vi "Get busy.vi"(8 "error in (no error)":errorcluster, 11 "Retiga in":refnum<class "Retiga.lvclass">) -> (0 "error out":errorcluster, 2 "busy?":bool, 3 "Retiga out":refnum<class "Retiga.lvclass">)   [LabVIEW 2012, in "Retiga.lvclass"]
uses:
  Retiga.lvclass
  Retiga.lvclass/Retiga.ctl
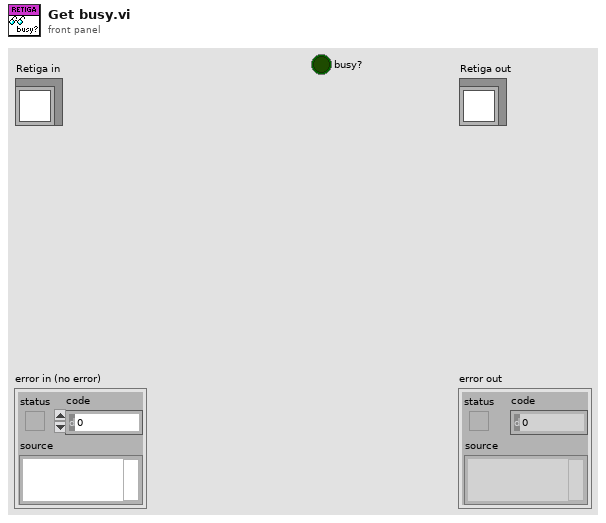
[diagram p1: front panel]
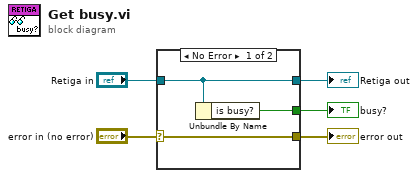
[diagram p0: block diagram]
diagram:
  n1 = case shown="No Error" "error in (no error)" {
    selector: "error in (no error)" -> [w8 w10]
    tunnel: [w8 w10] -> w4
    tunnel: [w7 w9] -> w2
    tunnel: "Retiga in" -> [w7 w9]
    tunnel: [w6 _] -> w1
    frame No Error {
      n2 = Unbundle By Name(w7) -> ("is busy?"=w6:bool)
    }
    frame Error {
    }
  }
  "error out" <- w4
  "Retiga out" <- w2
  "busy?" <- w1
